vi "Update Inst Config.vi"(8 "error in (no error)":errorcluster, 11 "Data In":string[](array[string])) -> (0 "error out":errorcluster, 3 "Scope":T1={"Connection"={"Ref"=variant}, "Channel Setting"={"Channel Name (0: Channel 1)"=0, "Coupling (1: DC)"=1, "Vertical Offset (0.0)"=0.0, "Vertical Range (40.0 V)"=40.0, "Probe Attenuation (1.0)"=1.0, "Enable Channel (T: Enable)"=TRUE, "Impedance (0: 1 MOhm)"=0, "Vertical Scale (5.0 V)"=5.0, "Vertical Setting (1: Vertical Range)"=1}} {"Channel Setting"."Vertical Setting (1: Vertical Range)" items=["Vertical Scale", "Vertical Range"]; "Channel Setting"."Impedance (0: 1 MOhm)" items=["1 MOhm", "50 Ohm"]; "Channel Setting"."Coupling (1: DC)" items=["AC", "DC"]; "Channel Setting"."Channel Name (0: Channel 1)" items=["Channel 1", "Channel 2", "Channel 3", "Channel 4"]})   [LabVIEW 2021, in "Oscilloscope.lvlib"]
uses:
  Oscilloscope.lvlib
  Scope Config Setting.ctl
  User Interface/User Interface.lvlib
panel:
  in  "Coupling (1: DC)":i32(ring)=1 items=["AC", "DC"]
  in  "Vertical Setting (1: Vertical Range)":i32(ring)=1 items=["Vertical Scale", "Vertical Range"]
  in  "Vertical Scale (5.0 V)":dbl=5.0
  in  "Impedance (0: 1 MOhm)":i32(ring) items=["1 MOhm", "50 Ohm"]
  in  "Probe Attenuation (1.0)":dbl=1.0
  in  "Vertical Range (40.0 V)":dbl=40.0
  in  "Vertical Offset (0.0)":dbl
  in  "Channel Name (0: Channel 1)":i32(ring) items=["Channel 1", "Channel 2", "Channel 3", "Channel 4"]
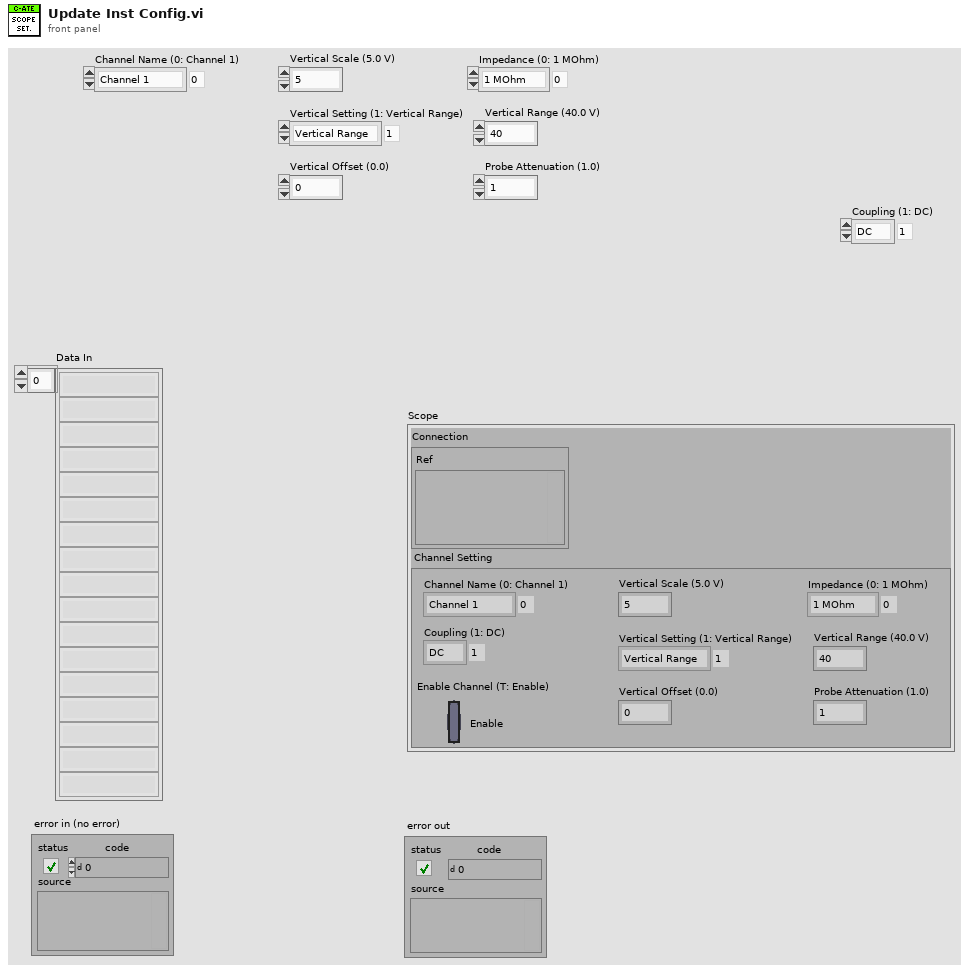
[diagram p1: front panel]
types:
  T1 = typedef "Oscilloscope.lvlib/Scope Config Setting.ctl" = cluster{"Connection":cluster{"Ref":variant}, "Channel Setting":cluster{"Channel Name (0: Channel 1)":i32, "Coupling (1: DC)":i32, "Vertical Offset (0.0)":dbl, "Vertical Range (40.0 V)":dbl, "Probe Attenuation (1.0)":dbl, "Enable Channel (T: Enable)":bool, "Impedance (0: 1 MOhm)":i32, "Vertical Scale (5.0 V)":dbl, "Vertical Setting (1: Vertical Range)":i32}}
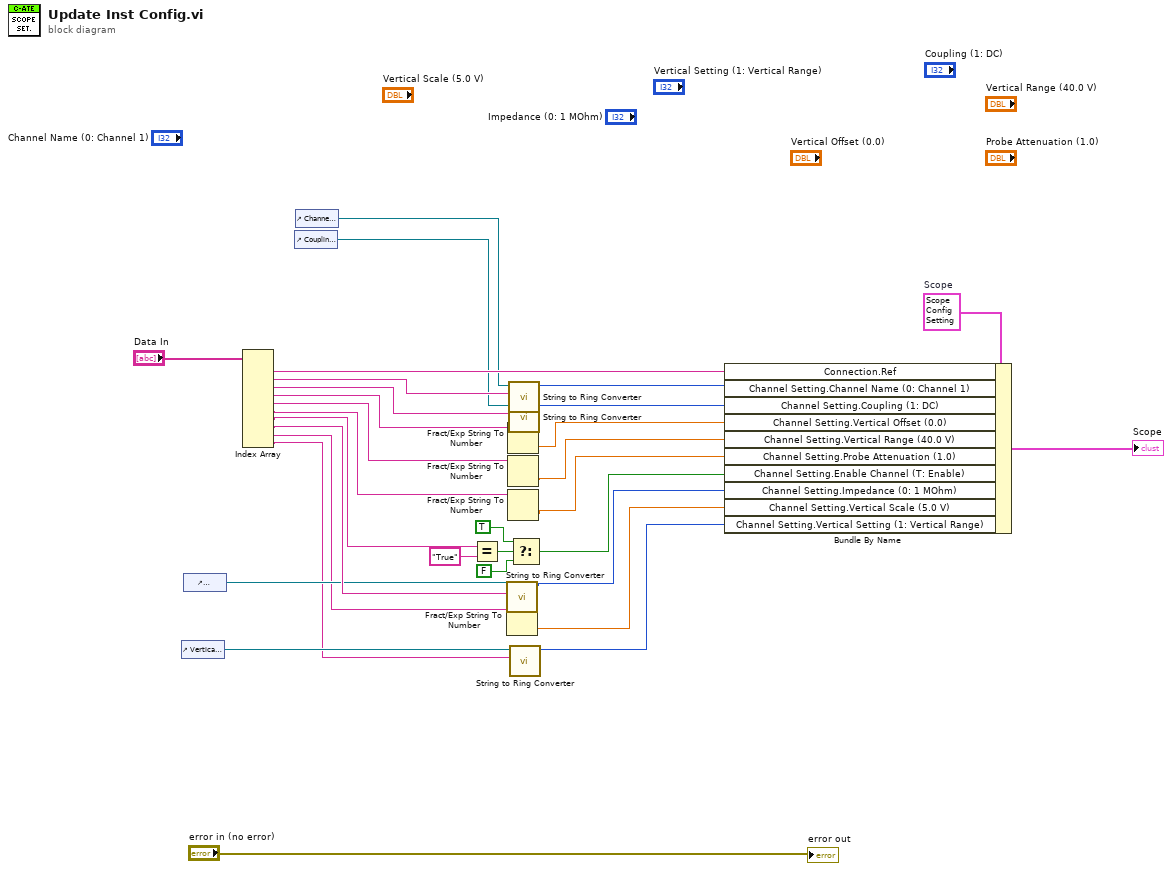
[diagram p0: block diagram]
diagram:
  w27 = T1 {"Connection"={"Ref"=variant}, "Channel Setting"={"Channel Name (0: Channel 1)"=0, "Coupling (1: DC)"=1, "Vertical Offset (0.0)"=0.0, "Vertical Range (40.0 V)"=40.0, "Probe Attenuation (1.0)"=1.0, "Enable Channel (T: Enable)"=TRUE, "Impedance (0: 1 MOhm)"=0, "Vertical Scale (5.0 V)"=5.0, "Vertical Setting (1: Vertical Range)"=1}}  # Scope
  n1 = control-ref of="Vertical Setting (1: Vertical Range)"() -> (w9:refnum<vi>)
  n2 = control-ref of="Impedance (0: 1 MOhm)"() -> (w13:refnum<vi>)
  n3 = Index Array(array="Data In") -> (element #1=w28:string, element #2=w25:string, element #3=w22:string, element #4=w20:string, element #5=w19:string, element #6=w18:string, element #7=w6:string, element #8=w14:string, element #9=w11:string, element #10=w8:string)  [unwired: 10 in]
  n4 = control-ref of="Coupling (1: DC)"() -> (w23:refnum<vi>)
  n5 = control-ref of="Channel Name (0: Channel 1)"() -> (w26:refnum<vi>)
  n6 = Equal?(x=w6, y="True") -> (x = y?=w4:bool)
  n7 = call "String to Ring Converter.vi"("Control Name"=w14, "Ring Control"=w13) -> ("Value"=w12:i32)  [unwired: 9 in]
  n8 = Fract/Exp String To Number(string=w11) -> (number=w10:dbl)  [unwired: 3 in, 1 out]
  n9 = Fract/Exp String To Number(string=w20) -> (number=w17:dbl)  [unwired: 3 in, 1 out]
  n10 = Fract/Exp String To Number(string=w19) -> (number=w16:dbl)  [unwired: 3 in, 1 out]
  n11 = Fract/Exp String To Number(string=w18) -> (number=w15:dbl)  [unwired: 3 in, 1 out]
  n12 = call "String to Ring Converter.vi"("Control Name"=w25, "Ring Control"=w26) -> ("Value"=w24:i32)  [unwired: 9 in]
  n13 = call "String to Ring Converter.vi"("Control Name"=w22, "Ring Control"=w23) -> ("Value"=w21:i32)  [unwired: 9 in]
  n14 = call "String to Ring Converter.vi"("Control Name"=w8, "Ring Control"=w9) -> ("Value"=w7:i32)  [unwired: 9 in]
  n15 = Select(t=TRUE, s=w4, f=FALSE) -> (s? t:f=w1:bool)
  n16 = Bundle By Name(cluster=w27, "Connection.Ref"=w28, "Channel Setting.Channel Name (0: Channel 1)"=w24, "Channel Setting.Coupling (1: DC)"=w21, "Channel Setting.Vertical Offset (0.0)"=w17, "Channel Setting.Vertical Range (40.0 V)"=w16, "Channel Setting.Probe Attenuation (1.0)"=w15, "Channel Setting.Enable Channel (T: Enable)"=w1, "Channel Setting.Impedance (0: 1 MOhm)"=w12, "Channel Setting.Vertical Scale (5.0 V)"=w10, "Channel Setting.Vertical Setting (1: Vertical Range)"=w7) -> (→"Scope":T1)
  "error out" <- "error in (no error)"
